vi "FEA_Model_Initialize_LEMP.vi"(11 "FEA_Model in":refnum<class "FEA_Model.lvclass">) -> (3 "FEA_Model out":refnum<class "FEA_Model.lvclass">)   [LabVIEW 2021, in "FEA_Model.lvclass"]
uses:
  FEA_Model.lvclass
  FEA_Model.lvclass/FEA_Model.ctl
  <vilib>/Analysis/Matrix/Numeric/Conversions/Matrix To Array - CM.vi
  <vilib>/Analysis/Matrix/NI_Matrix.lvlib
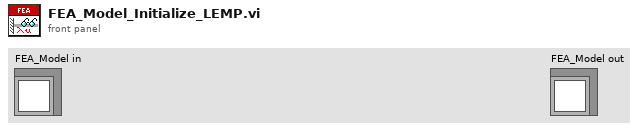
[diagram p1: front panel]
types:
  T1 = cluster{"Eigenvalues":dbl[], "Square Transpose Eigenvectors":dbl[][], "1/deltaStiff":dbl}
  T2 = enum16{"Particles to Nodes", "Particle to Node", "Nodes to Particles", "Node to Particle"}
  T3 = typedef "NI_Matrix.lvlib/ComplexMatrix.ctl" = cdb[][]
  T4 = enum16{"Scalar Particle to Meter", "Scalar Node to Meter", "Scalar Meter to Particle", "Scalar Meter to Node", "Array Particle to Meter", "Array Node to Meter", "Array Meter to Particle", "Array Meter to Node"}
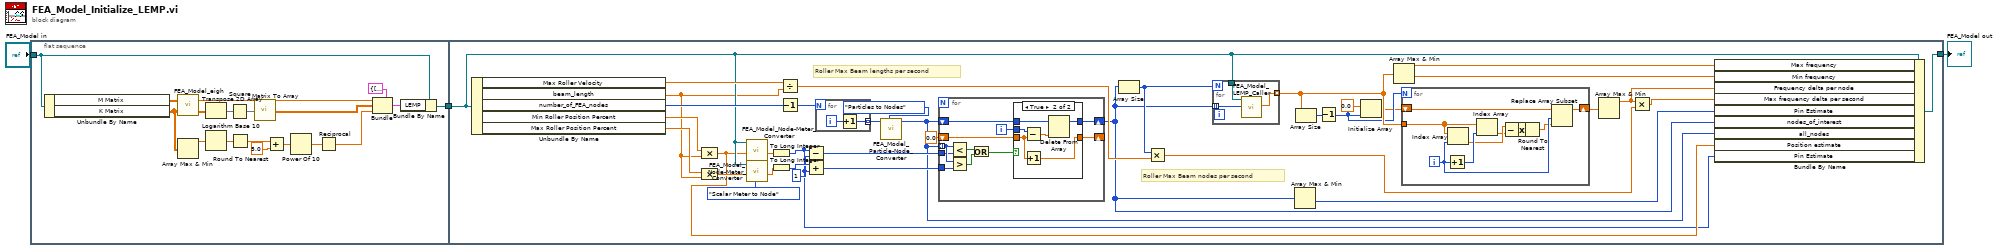
[diagram p0: block diagram]
diagram:
  n1 = flat-sequence {
    tunnel: "FEA_Model in" -> [w5]
    tunnel: [w4] -> w2
    tunnel: w2 -> [w36]
    tunnel: [w41] -> w1
    frame #0 {
      n2 = Unbundle By Name(w5) -> ("M Matrix"=w8:dbl[][], "K Matrix"=w7:dbl[][])
      n3 = call "FEA_Model_eigh.vi"("Stiffness"=w7, "Mass"=w8) -> ("Eigenvectors"=w13:T3, "Eigenvalues"=w11:dbl[])
      n4 = Array Max & Min(array=w7) -> (max value=w14:dbl)  [unwired: 3 out]
      n5 = Transpose 2D Array(2D array=w13) -> (transposed array=w21:T3)
      n6 = Logarithm Base 10(1:w14) -> (0:w17:dbl)
      n7 = Square(x=w21) -> (x^2=w20:T3)
      n8 = Round To Nearest(number=w17) -> (nearest integer value=w18:dbl)
      n9 = call-poly <vilib>:"Matrix To Array.vi"("Complex Matrix"=w20) -> ("Complex 2D Array"=w10:cdb[][])
      n10 = Add(x=w18, y=5.0) -> (x+y=w19:dbl)
      n11 = Power Of 10(x=w19) -> (10^x=w15:dbl)
      n12 = Reciprocal(x=w15) -> (1/x=w9:dbl)
      n13 = Bundle(cluster=T1 {"Eigenvalues"=[], "Square Transpose Eigenvectors"=[], "1/deltaStiff"=0.0} ("LEMP"), "Eigenvalues"=w11, "Square Transpose Eigenvectors"=w10, "1/deltaStiff"=w9) -> (w6:T1)
      n14 = Bundle By Name(cluster=w5, "LEMP"=w6) -> (w4:refnum<class "FEA_Model.lvclass">)
    }
    frame #1 {
      w29 = 1 ("y")
      w38 = T4."Scalar Meter to Node" ("Conversion Mode")
      # "Roller Max Beam nodes per second"
      # "Roller Max Beam lengths per second"
      n15 = Unbundle By Name(w36) -> ("Max Roller Velocity"=w44:dbl, "beam_length"=w28:dbl, "number_of_FEA_nodes"=w48:i32, "Min Roller Position Percent"=w39:dbl, "Max Roller Position Percent"=w40:dbl)
      n16 = Compound Arithmetic op=MULTIPLY(w39, w28) -> (w23:dbl)
      n17 = Compound Arithmetic op=MULTIPLY(w40, w28) -> (w37:dbl)
      n18 = call "FEA_Model_Node-Meter_Converter.vi"("Conversion Mode"=w38, "Scalar in"=w23, "FEA_Model in"=w36) -> ("Scalar out"=w35:dbl)  [unwired: 5 in, 3 out]
      n19 = call "FEA_Model_Node-Meter_Converter.vi"("Conversion Mode"=w38, "Scalar in"=w37, "FEA_Model in"=w36) -> ("Scalar out"=w34:dbl)  [unwired: 5 in, 3 out]
      n20 = To Long Integer(number=w35) -> (32bit integer=w22:i32)
      n21 = To Long Integer(number=w34) -> (32bit integer=w31:i32)
      n22 = Divide(x=w44, y=w28) -> (x/y=w42:dbl)
      n23 = Decrement(x=w48) -> (x-1=w33:i32)
      n24 = Subtract(x=w22, y=w29) -> (x-y=w32:i32)
      n25 = Add(x=w31, y=w29) -> (x+y=w30:i32)
      n26 = for {
        N: w33 -> [_]
        tunnel: [w91] -> w27 mode=indexing
        i -> [w92]
        n27 = Increment(x=w92) -> (x+1=w91:i32)
      }
      n28 = call "FEA_Model_Particle-Node_Converter.vi"("mode"=T2."Particles to Nodes", "Particles"=w27) -> ("Nodes"=w24:i32[])  [unwired: 6 in, 3 out]
      n29 = for {
        tunnel: w24 -> [w75] mode=indexing
        shift-right: [w78] -> w25
        shift-left: w24 -> [w82]
        shift-right: [w77] -> _
        shift-left: 0.0 -> [w76]
        tunnel: w32 -> [w73]
        tunnel: w30 -> [w72]
        i -> [w74]
        n30 = Less?(x=w75, y=w73) -> (x < y?=w79:bool)
        n31 = Greater?(x=w75, y=w72) -> (0:w81:bool)
        n32 = Or(x=w79, y=w81) -> (x .or. y?=w80:bool)
        n33 = case shown="True" w80 {
          tunnel: w82 -> [w84 w89]
          tunnel: [w84 w90] -> w78
          tunnel: [w83 w88] -> w77
          tunnel: w76 -> [w83 w87]
          tunnel: w74 -> [_ w86]
          frame False {
          }
          frame True {
            n34 = Subtract(x=w86, y=w87) -> (x-y=w85:dbl)
            n35 = Increment(x=w87) -> (x+1=w88:dbl)
            n36 = Delete From Array(array=w89, index=w85) -> (array with subset deleted=w90:i32[])  [unwired: 1 in, 1 out]
          }
        }
      }
      n37 = Array Size(array=w25) -> (size(s)=w47:i32)
      n38 = Multiply(x=w47, y=w42) -> (x*y=w43:dbl)
      n39 = for {
        N: w47 -> [_]
        tunnel: [w70] -> w57 mode=indexing
        tunnel: w25 -> [w69] mode=indexing
        tunnel: w36 -> [w71]
        n40 = call-dynamic "FEA_Model_LEMP_Caller.vi"("Node of interest"=w69, "FEA_Model in"=w71) -> ("Frequency"=w70:dbl)  [unwired: 7 in, 2 out]
      }
      n41 = Array Max & Min(array=w25) -> (min value=w58:i32)  [unwired: 3 out]
      n42 = Array Size(array=w57) -> (size(s)=w49:i32)
      n43 = Decrement(x=w49) -> (x-1=w52:i32)
      n44 = Initialize Array(0.0 ("element"), w52) -> (w50:dbl[])
      n45 = Array Max & Min(array=w57) -> (max value=w54:dbl, min value=w55:dbl)  [unwired: 2 out]
      n46 = for {
        N: w52 -> [_]
        tunnel: w57 -> [w68]
        shift-right: [w62] -> w53
        shift-left: w50 -> [w63]
        i -> [w61]
        n47 = Increment(x=w61) -> (x+1=w67:i32)
        n48 = Index Array(array=w68, index=w61) -> (element=w66:dbl)
        n49 = Index Array(array=w68, index=w67) -> (element=w65:dbl)
        n50 = Subtract(x=w66, y=w65) -> (x-y=w64:dbl)
        n51 = Absolute Value(x=w64) -> (abs(x)=w59:dbl)
        n52 = Round To Nearest(number=w59) -> (nearest integer value=w60:dbl)
        n53 = Replace Array Subset(array=w63, new element=w60, index=w61) -> (w62:dbl[])
      }
      n54 = Array Max & Min(array=w53) -> (max value=w56:dbl)  [unwired: 3 out]
      n55 = Multiply(x=w56, y=w43) -> (x*y=w45:dbl)
      n56 = Bundle By Name(cluster=w36, "Max frequency"=w54, "Min frequency"=w55, "Frequency delta per node"=w56, "Max frequency delta per second"=w45, "Pin Estimate"=w58, "nodes_of_interest"=w25, "all_nodes"=w24, "Position estimate"=w23, "Pin Estimate"=w22) -> (w41:refnum<class "FEA_Model.lvclass">)
    }
  }
  "FEA_Model out" <- w1
